vi "DisplayMessage.vi"(8 "error in (no error)":errorcluster, 11 "Message":string) -> ()   [LabVIEW 2013]
doc: "Create a pop-up window to display given message or error source.\n\nA window will not be created if there is no message and no error source."
panel:
  in  "OK":bool
  out "Display":string
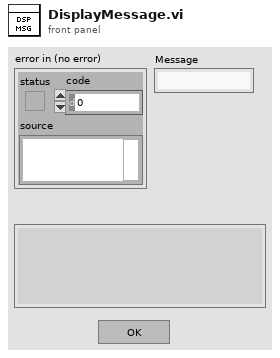
[diagram p1: front panel]
types:
  T1 = enum32{"Invalid", "Standard", "Closed", "Hidden", "Minimized", "Maximized"}
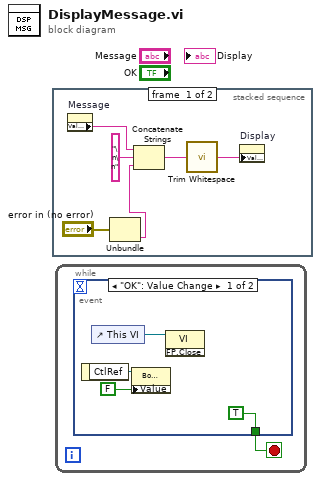
[diagram p0: block diagram]
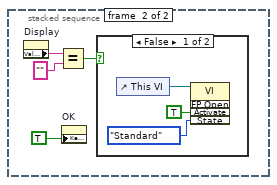
[diagram p2: hidden frame]
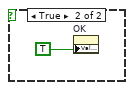
[diagram p3: hidden frame]
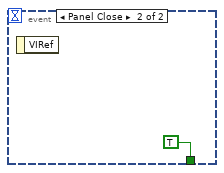
[diagram p4: hidden frame]
diagram:
  n1 = stacked-sequence {
    frame #0 {
      n2 = property on="Message" class="Str"() -> ("Value"=w3:string)  [unwired: 2 in, 2 out]
      n3 = Unbundle("error in (no error)") -> ("source"=w5:string)  [unwired: 2 out]
      n4 = Concatenate Strings(w3, "\n\n", w5) -> (w4:string)
      n5 = call <vilib>:"Trim Whitespace.vi"("string"=w4) -> ("trimmed string"=w1:string)  [unwired: 1 in]
      n6 = property on="Display" class="Str"("Value"=w1) -> ()  [unwired: 2 in, 2 out]
    }
    frame #1 {
      n7 = property on="Display" class="Str"() -> ("Value"=w10:string)  [unwired: 2 in, 2 out]
      n8 = Equal?(x=w10, y="") -> (x = y?=w8:bool)
      n9 = property on="OK" class="Bool (strict)"("Key Focus"=TRUE ("Activate?")) -> ()  [unwired: 2 in, 2 out]
      n10 = case shown="False" w8 {
        frame False {
          n11 = control-ref of="This VI"() -> (w13:refnum<vi>)
          n12 = invoke class="VI" method="FP.Open"(reference=w13, "Activate"=TRUE ("Activate?"), "State"=T1."Standard") -> ()  [unwired: 2 in, 5 out]
        }
        frame True {
          n13 = property on="OK" class="Bool (strict)"("Val(Sgnl)"=TRUE) -> ()  [unwired: 2 in, 2 out]
        }
      }
    }
  }
  n14 = while {
    stop <- w15 stop-if-true
    n15 = event shown="[0] \"OK\": Value Change" {
      selector: _ -> [_ _]
      dyn-events: _ -> [_ _]
      timeout: _ -> [_ _]
      tunnel: [TRUE TRUE] -> w15
      event "OK": Value Change {
        n16 = event-data() -> ("CtlRef"=w19:refnum<vi>)  [unwired: 1 in]
        n17 = control-ref of="This VI"() -> (w17:refnum<vi>)
        n18 = property class="Bool (strict)"(reference=w19, "Value"=FALSE) -> ()  [unwired: 1 in, 2 out]
        n19 = invoke class="VI" method="FP.Close"(reference=w17) -> ()  [unwired: 2 in, 3 out]
      }
      event Panel Close {
        n20 = event-data() -> ()  [unwired: 1 in, 1 out]
      }
    }
  }
